vi "z-stack acquistion.vi"() -> ()   [LabVIEW 2014]
uses:
  Globals/Initilize Globals.vi
  Stage Control/Stage SubVis/ctts/move stage.ctl
  File Directory/File-Locations-Global.vi
  Shutter Control/Shutter SubVis/ctts/control shutters.ctl
  <vilib>/vision/Image Controls.llb/IMAQ Image.ctl
  Glimpse-master/Glimpse core/Seq file v 1/Offset.ctl
  Glimpse-master/Glimpse core/Seq file v 1/file number.ctl
  Glimpse-master/Glimpse core/Seq file v 1/Offset table.ctl
  SubVIs/ctt's/Video acquisition state1.ctl
  SubVIs/ctt's/Image size and binning.ctl
  SubVIs/ctt's/Camera Setup Acquisition.ctl
  Shutter Control/Shutter SubVis/ctts/laser shutters.ctl
  SubVIs/ctt's/acquisition protocol z-stack.ctl
panel:
  in  "Acquisition Protocol":T1[](array[typedef])
  in  "Acquisition directory root path":path=path "c:/scratch"
  in  "stack half-width":u32
  in  "focus step (um)":dbl
  in  "Max. number of acquisition files":i8(slide)=10 scale=0.0..50.0
  in  "Cycle Interval (s)":dbl format="%_3f"
  in  "Image Size":T3={"H Bin"=1.0, "V Bin"=1.0, "Left"=1.0, "Right"=1024.0, "Top"=1.0, "Bottom"=1024.0} {"V Bin" min=0.0; "H Bin" min=0.0 step=1.0}
  in  "Acquisition Parameters":T4={"Readout Mode"=enum."Image", "Set Acquisition Mode"=enum."Single Scan", "Trigger Mode"=enum."Internal", "Exposure Time (sec)"=1.0, "Accumulation Cycle (s)"=1.0, "Kinetic Cycle Time (s)"=1.0, "Number of Kinetics"=1, "Number of Accumulations"=1, "Set VS Speed"=1.0, "Pixel Rate"=enum."Standard CCD 3 Mhz 14 bits", "V Shift Amplitude"=enum."+1", "Preamp Gain"=enum."1.0", "Single Track Settings"={"centre"=0, "height"=1}, "EM CCD Gain"=300, "High Capacity?"=FALSE} {"EM CCD Gain" scale=0.01..300.0; "Single Track Settings"."centre" min=0 max=1024; "Single Track Settings"."height" min=1 max=1024; "Exposure Time (sec)" scale=0.001..10.0 scale format="%#_1g"; "Set VS Speed" min=0.0 format="%#_2f"}
  # "Z-stack parameters"
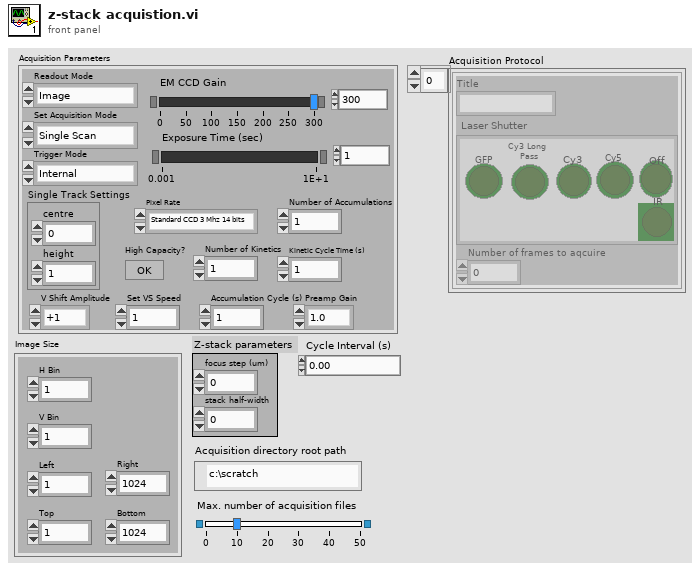
[diagram p1: front panel]
types:
  T1 = typedef "acquisition protocol z-stack.ctl" = cluster{"Title":string, "Laser Shutter":T2, "Number of frames to aqcuire":dbl}
  T2 = typedef "laser shutters.ctl" = enum32{"No Selection", "GFP", "Cy3 Long \nPass", "Cy3", "Cy5", "Off", "IR"}
  T3 = typedef "Image size and binning.ctl" = cluster{"H Bin":dbl, "V Bin":dbl, "Left":dbl, "Right":dbl, "Top":dbl, "Bottom":dbl}
  T4 = typedef "Camera Setup Acquisition.ctl" = cluster{"Readout Mode":enum16{"Full Vertical Binning", "Multi-Track", "Random-Track", "Single-Track", "Image"}, "Set Acquisition Mode":enum16{"(do nothing)", "Single Scan", "Accumulate", "Kinetics", "Fast Kinetics", "Run till abort"}, "Trigger Mode":enum16{"Internal", "External"}, "Exposure Time (sec)":sgl, "Accumulation Cycle (s)":dbl, "Kinetic Cycle Time (s)":dbl, "Number of Kinetics":i32, "Number of Accumulations":i32, "Set VS Speed":dbl, "Pixel Rate":enum16{"EM CCD 10 Mhz 14 bits", "EM CCD 5 Mhz 14 bits", "EM CCD 3 Mhz 14 bits", "EM CCD 1 Mhz 16 bits", "Standard CCD 3 Mhz 14 bits", "Standard CCD 1 Mhz 16 bits"}, "V Shift Amplitude":enum16{"normal", "+1", "+2", "+3", "+4"}, "Preamp Gain":enum16{"1.0", "2.4", "5.0"}, "Single Track Settings":cluster{"centre":i32, "height":i32}, "EM CCD Gain":u16, "High Capacity?":bool}
  T5 = cluster{"Frame Size (bytes)":i32, "Max Time (min)":i32, "Max Frames":i32, "Frames per acquisition file":i32, "Max time (s)":i32, "Max Space Req'd. (Gb)":dbl}
  T6 = typedef "acquisition control.ctl" = cluster{"H Bin":dbl, "V Bin":dbl, "Left":dbl, "Right":dbl, "Top":dbl, "Bottom":dbl}
  T7 = typedef "Video acquisition state1.ctl" = cluster{"Pixel depth":enum32{"8 bits", "16 bits", "Float", "Complex", "RGB Chunky", "Compressed"}, "Width":dbl, "Height":dbl, "Buffer":T8, "Frames Acquired":u32, "Time of 1st frame":dbl, "TTB element zero":u32, "File Offsets Array":T9, "TTB Array":u32[], "Sum Image (for averaging)":T8, "Time at end of last acquisition (ms)":u32, "Flow rate array":dbl[], "Temperature array":dbl[], "Field array":u16[], "Stage xyz array":dbl[][], "Current Filter Wheel Array":string[], "Laser Shutter Array":enum32{"No Selection", "GFP", "Cy3 Long \nPass", "Cy3", "Cy5", "Off", "IR"}[]}
  T8 = typedef "IMAQ Image.ctl" = refnum<image>
  T9 = typedef "Offset table.ctl" = cluster{"offset":T10, "file number":T11}[]
  T10 = typedef "Offset.ctl" = i32
  T11 = typedef "file number.ctl" = u8
  T12 = typedef "move stage.ctl" = cluster{"dx (um) (0 -> ignore)":ext, "dy (um) (0 -> ignore)":ext, "dz (um) (0 -> ignore)":ext, "Re-center x,y":bool, "Re-center z":bool, "x (um) (-1 -> ignore)":dbl, "y (um) (-1 -> ignore)":dbl, "z (um) (-1 -> ignore)":dbl}
  T13 = typedef "control shutters.ctl" = cluster{"Camera Shutter":bool, "Laser Shutter":enum32{"No Selection", "GFP", "Cy3 Long \nPass", "Cy3", "Cy5", "Off"}}
  T14 = enum32{"No Selection", "GFP", "Cy3 Long \nPass", "Cy3", "Cy5", "Off"}
  T15 = cluster{"Sequence files directory path":path, "Sequence files refnum array":refnum<file>[]}
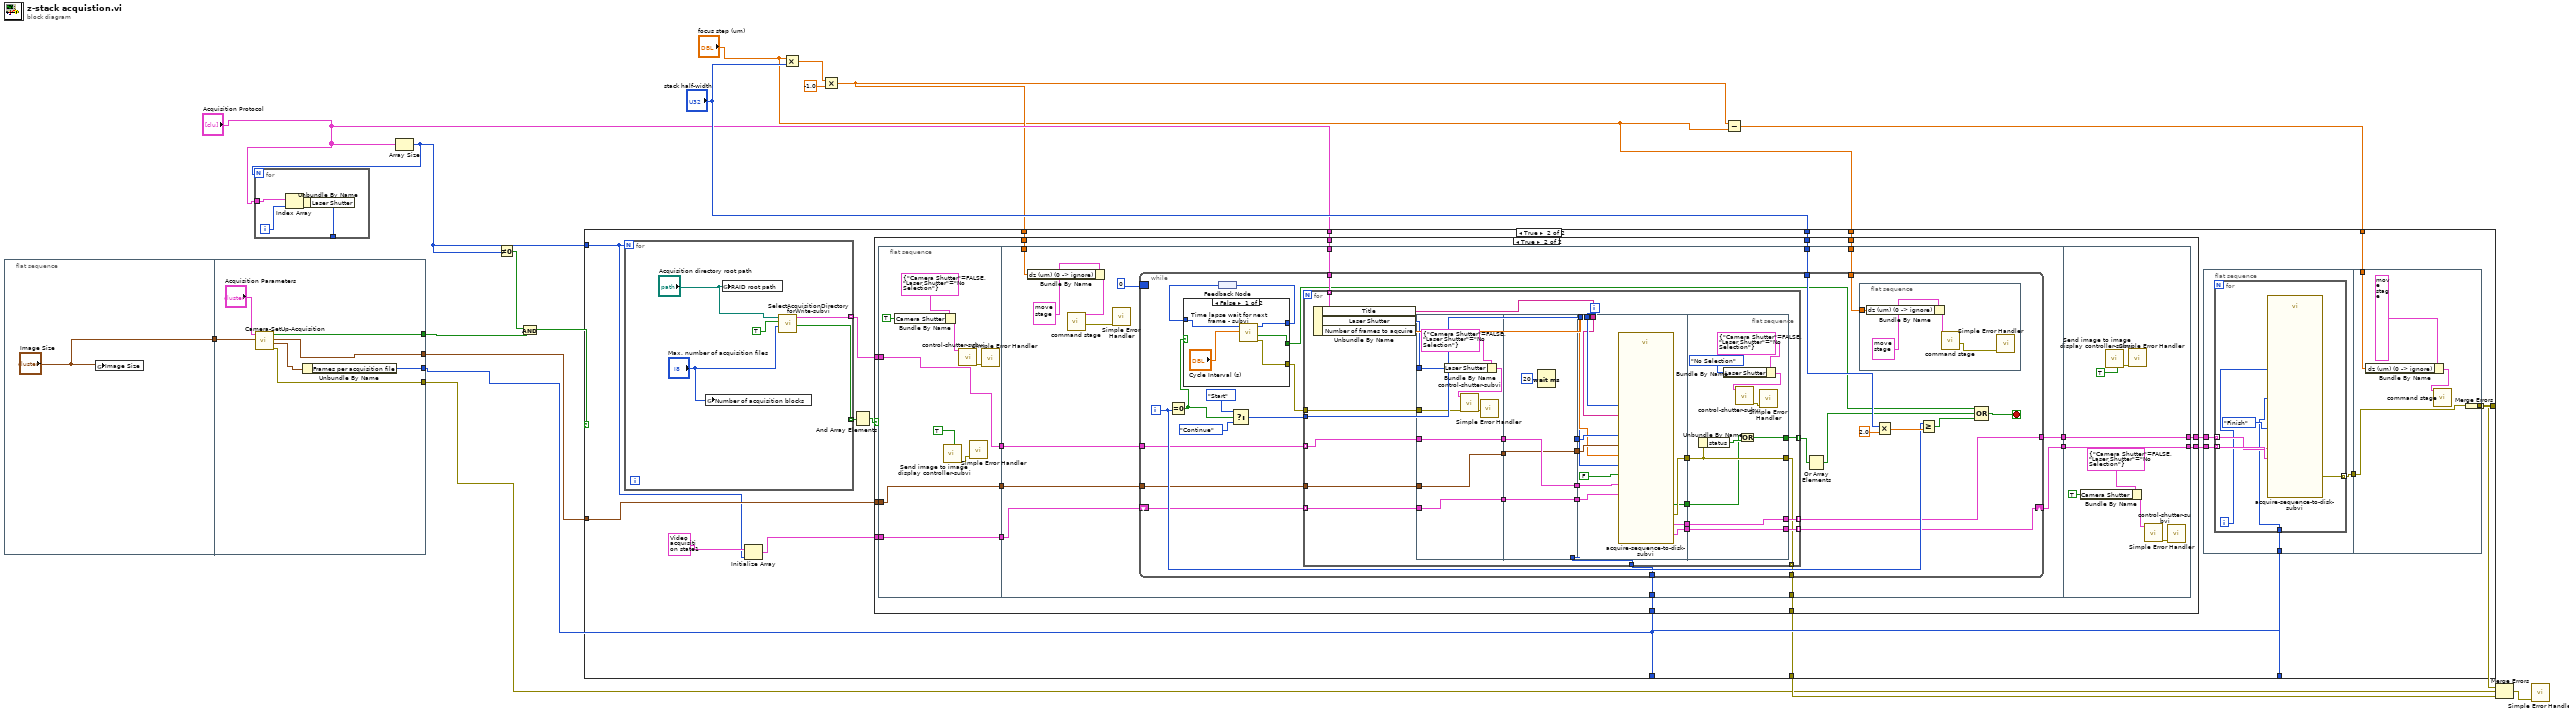
[diagram p0: block diagram]
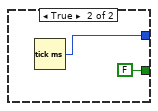
[diagram p4: hidden frame]
diagram:
  n1 = flat-sequence {
    tunnel: ["Image Size"] -> w19
    tunnel: w19 -> [w27]
    tunnel: [w25] -> w17
    tunnel: [w24] -> w4
    tunnel: [w23] -> w8
    tunnel: [w21] -> _
    tunnel: [w21] -> w10
    frame #0 {
      n2 = global write "Initilize Globals.vi" "Image Size"("Image Size") -> ()
    }
    frame #1 {
      n3 = call "Camera-SetUp-Acquisition.vi"("Image Size"=w27, "Acquisition Parameters"="Acquisition Parameters") -> ("Error Out"=w24:errorcluster, "File properties"=w22:T5, "Image Size Out"=w23:T6, "Continue with acq?"=w25:bool)  [unwired: 6 in]
      n4 = Unbundle By Name(w22) -> ("Frames per acquisition file"=w21:i32)
    }
  }
  n5 = Array Size(array="Acquisition Protocol") -> (size(s)=w13:i32)
  n6 = for {
    N: w13 -> [_]
    tunnel: "Acquisition Protocol" -> [w31]
    tunnel: [w28] -> _
    i -> [w30]
    n7 = Index Array(array=w31, index=w30) -> (element=w29:T1)
    n8 = Unbundle By Name(w29) -> ("Laser Shutter"=w28:T2)
  }
  n9 = Not Equal To 0?(x=w13) -> (x != 0?=w18:bool)
  n10 = And(x=w18, y=w17) -> (x .and. y?=w16:bool)
  n11 = Multiply(x="focus step (um)", y="stack half-width") -> (x*y=w15:dbl)
  n12 = Multiply(x=w15, y=-1.0) -> (x*y=w3:dbl)
  n13 = Subtract(x=w3, y="focus step (um)") -> (x-y=w1:dbl)
  n14 = case shown="True" w16 {
    tunnel: w13 -> [_ w39]
    tunnel: [_ w46] -> w12
    tunnel: "stack half-width" -> [_ w45]
    tunnel: w10 -> [_ w44]
    tunnel: w10 -> [_ w43]
    tunnel: "Acquisition Protocol" -> [_ w42]
    tunnel: w8 -> [_ w41]
    tunnel: [_ w35] -> w5
    tunnel: w3 -> [_ w34]
    tunnel: "focus step (um)" -> [_ w33]
    tunnel: w1 -> [_ w32]
    frame False {
    }
    frame True {
      n15 = for {
        N: w39 -> [_]
        tunnel: [w215] -> w49 mode=indexing
        tunnel: [w214] -> w48 mode=indexing
        n16 = global write "Initilize Globals.vi" "Number of acquisition blocks"("Max. number of acquisition files") -> ()
        n17 = global write "File-Locations-Global.vi" "RAID root path"("Acquisition directory root path") -> ()
        n18 = call "SelectAcquisitionDirectoryforWrite-subvi.vi"("Number of acquisition files"="Max. number of acquisition files", "Autostart?"=TRUE, "Acquisition directory root path"="Acquisition directory root path") -> ("OK?"=w215:bool, "Sequence files handle"=w214:T15)  [unwired: 7 in]
      }
      n19 = Initialize Array(T7 {"Pixel depth"=enum."8 bits", "Width"=0.0, "Height"=0.0, "Buffer"=refnum, "Frames Acquired"=0, "Time of 1st frame"=0.0, "TTB element zero"=0, "File Offsets Array"=[], "TTB Array"=[], "Sum Image (for averaging)"=refnum, "Time at end of last acquisition (ms)"=0, "Flow rate array"=[], "Temperature array"=[], "Field array"=[], "Stage xyz array"=[], "Current Filter Wheel Array"=[], "Laser Shutter Array"=[]} ("State"), w39) -> (w38:T7[])
      n20 = And Array Elements(Boolean array=w49) -> (logical AND=w50:bool)
      n21 = case shown="True" w50 {
        tunnel: w48 -> [w66 w78]
        tunnel: w45 -> [_ w82]
        tunnel: w44 -> [_ w81]
        tunnel: w42 -> [_ w80]
        tunnel: w41 -> [_ w77]
        tunnel: w38 -> [w65 w74]
        tunnel: [w65 w73] -> w37
        tunnel: [w66 w70] -> w36
        tunnel: [_ w69] -> w35
        tunnel: w34 -> [_ w68]
        tunnel: w33 -> [_ w67]
        frame False {
        }
        frame True {
          n22 = flat-sequence {
            tunnel: [w85] -> w79
            tunnel: w78 -> [w85]
            tunnel: w77 -> [w84]
            tunnel: [w84] -> w76
            tunnel: [w83] -> w75
            tunnel: w74 -> [w83]
            tunnel: w82 -> [w102]
            tunnel: w81 -> [w101]
            tunnel: w80 -> [w100]
            tunnel: w79 -> [w99]
            tunnel: w76 -> [w98]
            tunnel: w75 -> [w97]
            tunnel: [w96] -> w72
            tunnel: [w95] -> w71
            tunnel: [w94] -> w69
            tunnel: w68 -> [w93]
            tunnel: w67 -> [w92]
            tunnel: [w206] -> w73
            tunnel: w72 -> [w206]
            tunnel: w71 -> [w205]
            tunnel: [w205] -> w70
            frame #0 {
              n23 = Bundle By Name(cluster=T13 {"Camera Shutter"=FALSE, "Laser Shutter"=enum."No Selection"} ("Shutter Control"), "Camera Shutter"=TRUE) -> (w89:T13)
              n24 = call "Send image to image display controller-subvi.vi"("Start display controller?"=TRUE) -> ("error out"=w87:errorcluster)  [unwired: 8 in, 1 out]
              n25 = call "control-shutter-subvi.vi"("Shutter Control"=w89) -> ("Error Out"=w86:errorcluster)  [unwired: 10 in]
              n26 = call <vilib>:"Simple Error Handler.vi"("error in (no error)"=w87) -> ()  [unwired: 4 in, 5 out]
              n27 = call <vilib>:"Simple Error Handler.vi"("error in (no error)"=w86) -> ()  [unwired: 4 in, 5 out]
            }
            frame #1 {
              n28 = Bundle By Name(cluster=T12 {"dx (um) (0 -> ignore)"=0.0, "dy (um) (0 -> ignore)"=0.0, "dz (um) (0 -> ignore)"=0.0, "Re-center x,y"=FALSE, "Re-center z"=FALSE, "x (um) (-1 -> ignore)"=-1.0, "y (um) (-1 -> ignore)"=-1.0, "z (um) (-1 -> ignore)"=-1.0} ("Command Stage"), "dz (um) (0 -> ignore)"=w93) -> (w104:T12)
              n29 = call "command stage.vi"("Command Stage"=w104) -> ("Error Out"=w106:errorcluster)  [unwired: 10 in]
              n30 = call <vilib>:"Simple Error Handler.vi"("error in (no error)"=w106) -> ()  [unwired: 4 in, 5 out]
              n31 = while {
                border: 0 -> [_]
                tunnel: w102 -> [w124]
                tunnel: w101 -> [w119]
                tunnel: w100 -> [w118]
                tunnel: w99 -> [w117]
                tunnel: w98 -> [w116]
                shift-right: [w110] -> w96
                shift-left: w97 -> [w115]
                tunnel: [w109] -> w95
                tunnel: [w108] -> w94
                tunnel: w92 -> [w107]
                i -> [w125]
                stop <- w129 stop-if-true
                n32 = Equal To 0?(x=w125) -> (x = 0?=w123:bool)
                n33 = feedback #1() -> (w130:u32)
                n34 = case shown="False" w123 {
                  tunnel: [w197 _] -> w114
                  tunnel: [w196 FALSE ("Stopped?")] -> w111
                  tunnel: [w195 w200] -> w131
                  tunnel: w130 -> [w194 _]
                  frame False {
                    n35 = call "Time lapse wait for next frame - subvi.vi"("Frame Interval (s)"="Cycle Interval (s)", "Time of last frame in"=w194) -> ("Error Out"=w197:errorcluster, "Stopped?"=w196:bool, "Time of this frame out (ms)"=w195:i32)  [unwired: 6 in, 1 out]
                  }
                  frame True {
                    n36 = Tick Count (ms)() -> (millisecond timer value=w200:u32)
                  }
                }
                n37 = feedback-in #1(w131) -> ()
                n38 = Select(t=enum16{"Start", "Continue", "Finish"}."Start" ("Operation"), s=w123, f=enum16{"Start", "Continue", "Finish"}."Continue" ("Operation")) -> (s? t:f=w120:enum16{"Start", "Continue", "Finish"})
                n39 = for {
                  tunnel: w120 -> [w142]
                  tunnel: w119 -> [w146]
                  tunnel: w118 -> [w157] mode=indexing
                  tunnel: w117 -> [w155] mode=indexing
                  tunnel: w116 -> [w153]
                  tunnel: w115 -> [w150] mode=indexing
                  tunnel: w114 -> [w141]
                  tunnel: [w137] -> w113 mode=indexing
                  tunnel: [w135] -> w110 mode=indexing
                  tunnel: [w134] -> w109 mode=indexing
                  tunnel: [w132] -> w108 mode=indexing
                  i -> [w145]
                  n40 = Unbundle By Name(w157) -> ("Title"=w144:string, "Laser Shutter"=w140:T2, "Number of frames to aqcuire"=w143:dbl)
                  n41 = flat-sequence {
                    tunnel: [w165] -> w156
                    tunnel: w155 -> [w165]
                    tunnel: w153 -> [w164]
                    tunnel: [w164] -> w151
                    tunnel: w150 -> [w163]
                    tunnel: [w163] -> w148
                    tunnel: w141 -> [w162]
                    tunnel: w140 -> [w160]
                    tunnel: w156 -> [w170]
                    tunnel: [w170] -> w154
                    tunnel: [w169] -> w152
                    tunnel: w151 -> [w169]
                    tunnel: [w168] -> w149
                    tunnel: w148 -> [w168]
                    tunnel: [w167] -> w147
                    tunnel: w146 -> [w167]
                    tunnel: w154 -> [w181]
                    tunnel: w152 -> [w182]
                    tunnel: w149 -> [w180]
                    tunnel: w147 -> [w179]
                    tunnel: w145 -> [w178]
                    tunnel: w144 -> [w177]
                    tunnel: w143 -> [w176]
                    tunnel: w142 -> [w175]
                    tunnel: [w174] -> w139
                    tunnel: [w173] -> w138
                    tunnel: [w172] -> w136
                    tunnel: [w171] -> w133
                    tunnel: [w189] -> w132
                    tunnel: w139 -> [w189]
                    tunnel: w138 -> [w187]
                    tunnel: [w186] -> w137
                    tunnel: [w185] -> w135
                    tunnel: w136 -> [w185]
                    tunnel: [w184] -> w134
                    tunnel: w133 -> [w184]
                    frame #0 {
                      n42 = Bundle By Name(cluster=T13 {"Camera Shutter"=FALSE, "Laser Shutter"=enum."No Selection"} ("Shutter Control"), "Laser Shutter"=w160) -> (w159:T13)
                      n43 = call "control-shutter-subvi.vi"("Error In"=w162, "Shutter Control"=w159) -> ("Error Out"=w158:errorcluster)  [unwired: 9 in]
                      n44 = call <vilib>:"Simple Error Handler.vi"("error in (no error)"=w158) -> ()  [unwired: 4 in, 5 out]
                    }
                    frame #1 {
                      n45 = Wait (ms)(milliseconds to wait=u32 20) -> ()  [unwired: 1 out]
                    }
                    frame #2 {
                      n46 = call "acquire-sequence-to-disk-subvi.vi"("Image Size"=w182, "Operation"=w175, "Number of frames to acquire"=w176, "State In"=w180, "Frames per acquisition file"=w179, "Sequence files handle"=w181, "Pressing stop \nautomatically runs finish?"=FALSE ("Pressing stop \nautomatically runs finish?"), "Display Window Title"=w177, "Display Window Number"=w178) -> ("Done?"=w173:bool, "State Out"=w172:T7, "Sequence files handle out"=w171:T15, "Error Out"=w174:errorcluster)  [unwired: 3 in]
                    }
                    frame #3 {
                      n47 = Unbundle By Name(w189) -> ("status"=w188:bool)
                      n48 = Bundle By Name(cluster=T13 {"Camera Shutter"=FALSE, "Laser Shutter"=enum."No Selection"} ("Shutter Control"), "Laser Shutter"=T14."No Selection") -> (w191:T13)
                      n49 = call "control-shutter-subvi.vi"("Shutter Control"=w191) -> ("Error Out"=w190:errorcluster)  [unwired: 10 in]
                      n50 = Or(x=w187, y=w188) -> (x .or. y?=w186:bool)
                      n51 = call <vilib>:"Simple Error Handler.vi"("error in (no error)"=w190) -> ()  [unwired: 4 in, 5 out]
                    }
                  }
                }
                n52 = Or Array Elements(Boolean array=w113) -> (logical OR=w112:bool)
                n53 = flat-sequence {
                  tunnel: w107 -> [w201]
                  frame #0 {
                    n54 = Bundle By Name(cluster=T12 {"dx (um) (0 -> ignore)"=0.0, "dy (um) (0 -> ignore)"=0.0, "dz (um) (0 -> ignore)"=0.0, "Re-center x,y"=FALSE, "Re-center z"=FALSE, "x (um) (-1 -> ignore)"=-1.0, "y (um) (-1 -> ignore)"=-1.0, "z (um) (-1 -> ignore)"=-1.0} ("Command Stage"), "dz (um) (0 -> ignore)"=w201) -> (w202:T12)
                    n55 = call "command stage.vi"("Command Stage"=w202) -> ("Error Out"=w204:errorcluster)  [unwired: 10 in]
                    n56 = call <vilib>:"Simple Error Handler.vi"("error in (no error)"=w204) -> ()  [unwired: 4 in, 5 out]
                  }
                }
                n57 = Multiply(x=w124, y=2.0) -> (x*y=w127:dbl)
                n58 = Greater Or Equal?(x=w125, y=w127) -> (x >= y?=w128:bool)
                n59 = Compound Arithmetic op=OR(w111, w112, w128) -> (w129:bool)
              }
            }
            frame #2 {
              n60 = Bundle By Name(cluster=T13 {"Camera Shutter"=FALSE, "Laser Shutter"=enum."No Selection"} ("Shutter Control"), "Camera Shutter"=TRUE) -> (w210:T13)
              n61 = call "Send image to image display controller-subvi.vi"("Quit display controller?"=TRUE) -> ("error out"=w207:errorcluster)  [unwired: 8 in, 1 out]
              n62 = call <vilib>:"Simple Error Handler.vi"("error in (no error)"=w207) -> ()  [unwired: 4 in, 5 out]
              n63 = call "control-shutter-subvi.vi"("Shutter Control"=w210) -> ("Error Out"=w209:errorcluster)  [unwired: 10 in]
              n64 = call <vilib>:"Simple Error Handler.vi"("error in (no error)"=w209) -> ()  [unwired: 4 in, 5 out]
            }
          }
        }
      }
      n65 = flat-sequence {
        tunnel: [w54] -> w47
        tunnel: w43 -> [w53]
        tunnel: w37 -> [w52]
        tunnel: w36 -> [w51]
        tunnel: w47 -> [w62]
        tunnel: [w62] -> w46
        tunnel: w32 -> [w61]
        frame #0 {
          n66 = for {
            tunnel: [w60] -> w54 mode=indexing
            tunnel: w53 -> [w55]
            tunnel: w52 -> [w58] mode=indexing
            tunnel: w51 -> [w57] mode=indexing
            i -> [w56]
            n67 = call "acquire-sequence-to-disk-subvi.vi"("Operation"=enum16{"Start", "Continue", "Finish"}."Finish", "State In"=w58, "Frames per acquisition file"=w55, "Sequence files handle"=w57, "Display Window Number"=w56) -> ("Error Out"=w60:errorcluster)  [unwired: 7 in, 3 out]
          }
        }
        frame #1 {
          n68 = Bundle By Name(cluster=T12 {"dx (um) (0 -> ignore)"=0.0, "dy (um) (0 -> ignore)"=0.0, "dz (um) (0 -> ignore)"=0.0, "Re-center x,y"=FALSE, "Re-center z"=FALSE, "x (um) (-1 -> ignore)"=-1.0, "y (um) (-1 -> ignore)"=-1.0, "z (um) (-1 -> ignore)"=-1.0} ("Command Stage"), "dz (um) (0 -> ignore)"=w61) -> (w63:T12)
          n69 = call "command stage.vi"("Command Stage"=w63) -> ()  [unwired: 10 in, 1 out]
        }
      }
    }
  }
  n70 = Merge Errors(w12) -> (w6:errorcluster)
  n71 = Merge Errors(w6, w4, w5) -> (w7:errorcluster)
  n72 = call <vilib>:"Simple Error Handler.vi"("error in (no error)"=w7) -> ()  [unwired: 4 in, 5 out]
